vi "CostEstimate.vi"() -> ()   [LabVIEW 2019]
panel:
  out "COST (LKR)":dbl[](array[numeric])=[100.0, 100.0, 100.0, 100.0, 150.0, 150.0, 100.0, 150.0, 100.0, 150.0]
  in  "Rate (LKR)":dbl=50.0
  out ">30m":bool[](array[boolean])=[TRUE, FALSE, FALSE, FALSE, TRUE, TRUE, FALSE, TRUE, FALSE, TRUE]
  out "s":i32[](array[numeric])=[49, 7, 38, 26, 8, 0, 35, 16, 55, 39]
  out "m":i32[](array[numeric])=[40, 19, 23, 6, 41, 45, 27, 30, 16, 30]
  out "h":i32[](array[numeric])=[1, 2, 2, 2, 2, 2, 2, 2, 2, 2]
  in  "Seconds":u64[](array[numeric])=[6049, 8347, 8618, 7586, 9668, 9900, 8855, 9016, 8215, 9039]
  out "Time string":string[](array[string])=["01:40:49", "02:19:07", "02:23:38", "02:06:26", "02:41:08", "02:45:00", "02:27:35", "02:30:16", "02:16:55", "02:30:39"]
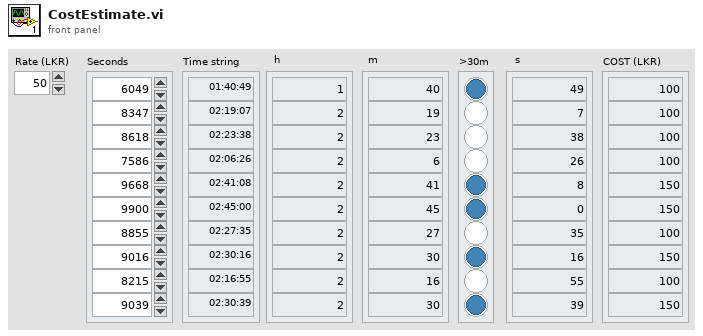
[diagram p1: front panel]
types:
  T1 = cluster{"Time String":string, "h":i32, "m":i32, ">30m":bool, "s":i32, "Cost":dbl}
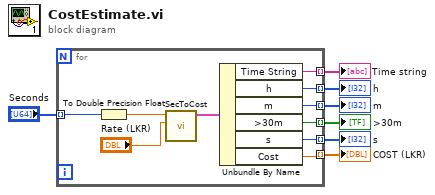
[diagram p0: block diagram]
diagram:
  n1 = for {
    tunnel: "Seconds" -> [w17] mode=indexing
    tunnel: [w13] -> w6 mode=indexing
    tunnel: [w12] -> w5 mode=indexing
    tunnel: [w11] -> w4 mode=indexing
    tunnel: [w9] -> w3 mode=indexing
    tunnel: [w10] -> w2 mode=indexing
    tunnel: [w8] -> w1 mode=indexing
    n2 = To Double Precision Float(number=w17) -> (double precision float=w15:dbl)
    n3 = call "SecToCost.vi"("Rate"="Rate (LKR)", "Seconds"=w15) -> ("StoCcluster"=w14:T1)  [unwired: 9 in]
    n4 = Unbundle By Name(w14) -> ("Time String"=w13:string, "h"=w12:i32, "m"=w11:i32, ">30m"=w10:bool, "s"=w9:i32, "Cost"=w8:dbl)
  }
  "Time string" <- w6
  "h" <- w5
  "m" <- w4
  "s" <- w3
  ">30m" <- w2
  "COST (LKR)" <- w1
